vi "DAQEG_DAQ DATA Queue FGV.vi"(6 "Command":enum16{"Initialize", "Get Value", "Set Value"}(ring)=enum."Get Value", 8 "error in":errorcluster, 11 "data queue[]":T1[](array[typedef])) -> (0 "error out":errorcluster, 3 "data queue[] out":T1[](array[typedef]))   [LabVIEW 2016]
uses:
  HardWare/Ctrls/HardWare _ Data Queue Info.ctl
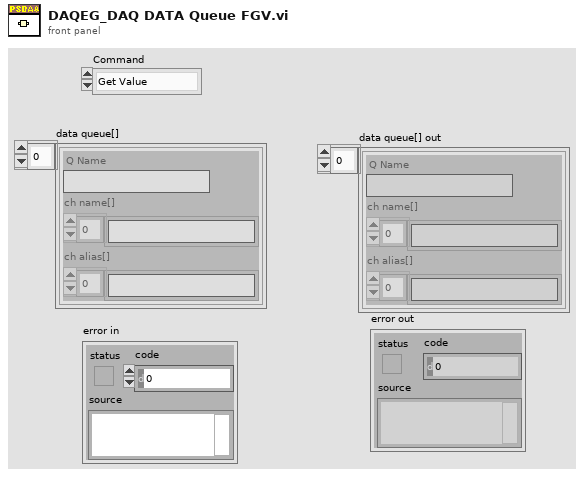
[diagram p1: front panel]
types:
  T1 = typedef "HardWare _ Data Queue Info.ctl" = cluster{"Q Name":string, "ch name[]":string[], "ch alias[]":string[]}
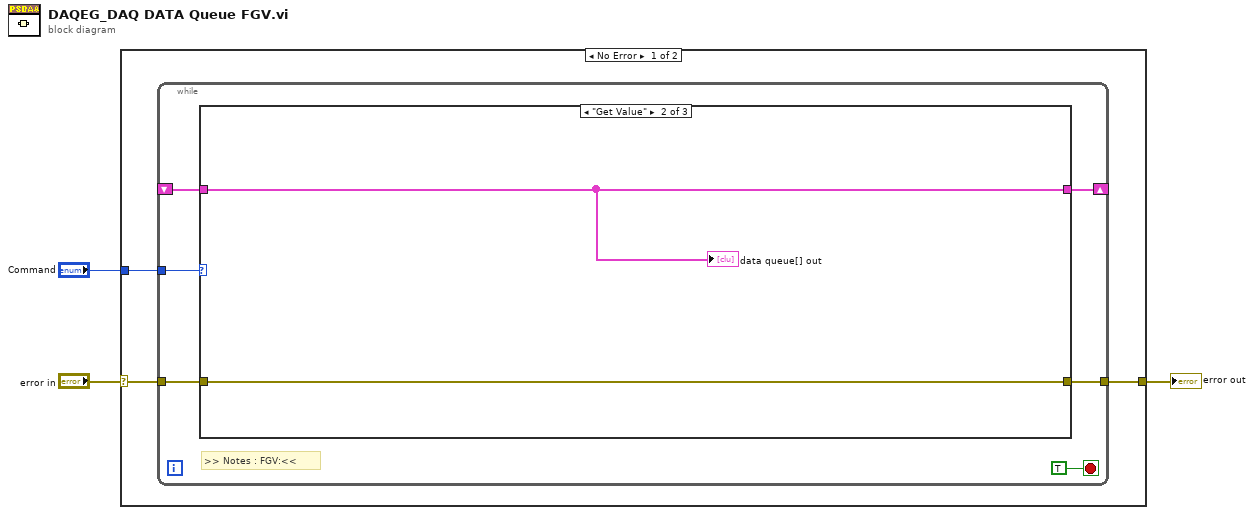
[diagram p0: block diagram]
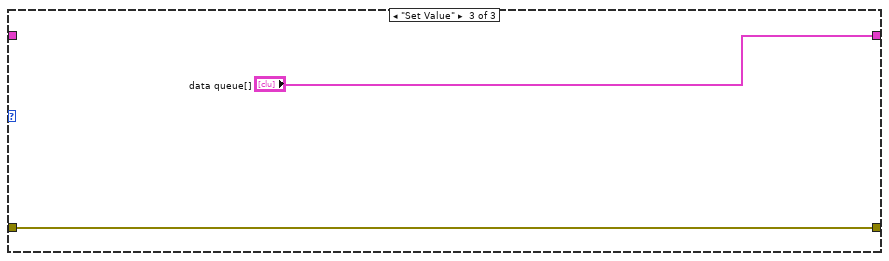
[diagram p3: hidden frame]
diagram:
  n1 = case shown="No Error" "error in" {
    selector: "error in" -> [w5 w18]
    tunnel: [w4 w18] -> w3
    tunnel: "Command" -> [w6 _]
    frame No Error {
      n2 = while {
        tunnel: w6 -> [w11]
        tunnel: w5 -> [w10]
        tunnel: [w9] -> w4
        shift-right: [w8] -> _
        shift-left: _ -> [w7]
        stop <- TRUE stop-if-true
        # ">> Notes : FGV:<<"
        n3 = case shown="\"Get Value\"" w11 {
          tunnel: w10 -> [w13 w15 w17]
          tunnel: [w13 w15 w17] -> w9
          tunnel: [_ w14 "data queue[]"] -> w8
          tunnel: w7 -> [_ w14 _]
          frame "Initialize", Default {
          }
          frame "Get Value" {
            "data queue[] out" <- w14
          }
          frame "Set Value" {
          }
        }
      }
    }
    frame Error {
    }
  }
  "error out" <- w3
